vi "Copy Definition.vi"(4 "Parent Linked List ID":string, 6 "Linked List ID":string, 7 "Linked List Definition Source":refnum<class "Linked List Definition.lvclass">, 10 "Child IDs":string[](array[string]), 11 "Linked List Definition in":refnum<class "Linked List Definition.lvclass">) -> (3 "Linked List Definition out":refnum<class "Linked List Definition.lvclass">)   [LabVIEW 2017, in "Linked Lists.lvlib" / "Linked List Definition.lvclass"]
uses:
  <vilib>/gpm_packages/@cs/linked-list/Source/Linked List/Linked List Definition/Linked List Definition.lvclass
  <vilib>/gpm_packages/@cs/linked-list/Source/Linked List/Linked List Definition/Linked List Definition.lvclass/Linked List Definition.ctl
  <vilib>/gpm_packages/@cs/linked-list/Source/Linked List/Linked List Header/Linked List Header.lvclass
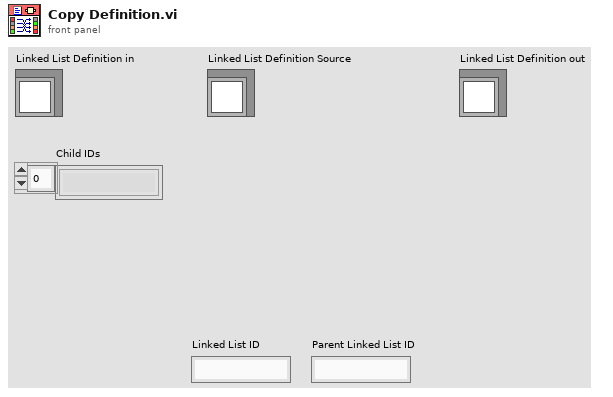
[diagram p1: front panel]
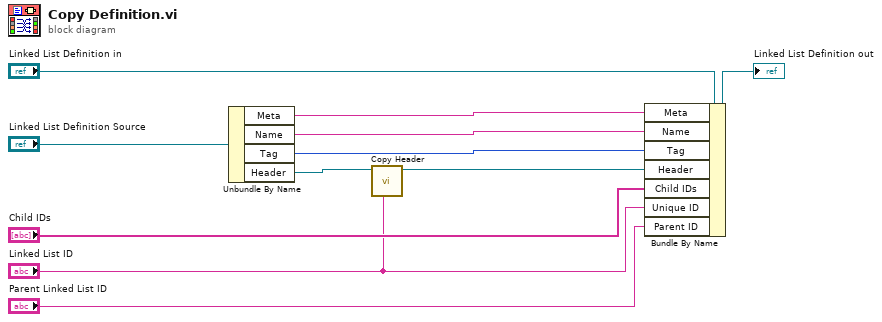
[diagram p0: block diagram]
diagram:
  n1 = Unbundle By Name("Linked List Definition Source") -> ("Meta"=w4:string, "Name"=w8:string, "Tag"=w7:i8, "Header"=w3:refnum<class "Linked List Header.lvclass">)
  n2 = call <vilib>:"Copy Header.vi"("GUID"="Linked List ID", "Linked List Header in"=w3) -> ("Linked List Header out"=w1:refnum<class "Linked List Header.lvclass">)  [unwired: 8 in, 1 out]
  n3 = Bundle By Name(cluster="Linked List Definition in", "Meta"=w4, "Name"=w8, "Tag"=w7, "Header"=w1, "Child IDs"="Child IDs", "Unique ID"="Linked List ID", "Parent ID"="Parent Linked List ID") -> (→"Linked List Definition out":refnum<class "Linked List Definition.lvclass">)
